vi "SDO_TRAJECTORY_EXECUTE_REL.vi"(8 "Init":bool, 10 "End Relative\nOrientation Deg":dbl, 11 "Gyro Heading\nRAD":dbl) -> (0 "AtReference":bool, 3 "Chassis Velocity Target":T1 {"vOmega" format="%10.3f"; "vY" format="%10.3f"; "vX" format="%10.3f"})   [LabVIEW 2019]
uses:
  <vilib>/Rock Robotics/WPI/ThirdParty/JAS_Junk/TrajLib/Trajectory_Library.lvlib
  PPS_TRAJECTORY_GLOBALS.vi
  <vilib>/Rock Robotics/WPI/ThirdParty/JAS_Junk/TrajLib/TypeDef/CHASSIS_SPEEDS.ctl
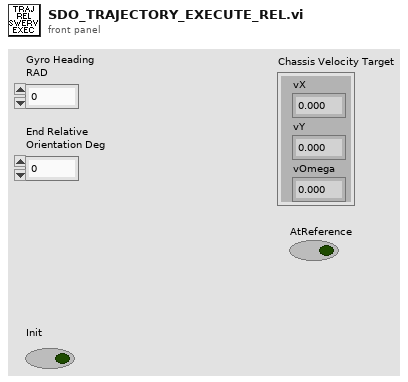
[diagram p1: front panel]
types:
  T1 = typedef "Trajectory_Library.lvlib/CHASSIS_SPEEDS.ctl" = cluster{"vX":dbl, "vY":dbl, "vOmega":dbl}
  T2 = typedef "Trajectory_Library.lvlib/ROTATION2D.ctl" = cluster{"VALUE":dbl, "COS":dbl, "SIN":dbl}
  T3 = typedef "Trajectory_Library.lvlib/SWERVE_DRIVE_KINEMATICS.ctl" = cluster{"NumModules":i32, "InverseKinematics":T4, "ForwardKinematics":T4, "Modules":T5[], "PrevCoR":T5, "SavedModuleStates":T6[]}
  T4 = typedef "NI_Matrix.lvlib/RealMatrix.ctl" = dbl[][]
  T5 = typedef "Trajectory_Library.lvlib/TRANSLATION2D.ctl" = cluster{"X":dbl, "Y":dbl}
  T6 = typedef "Trajectory_Library.lvlib/SWERVE_DRIVE_MODULE_STATE.ctl" = cluster{"Speed":dbl, "Angle":T2}
  T7 = typedef "Trajectory_Library.lvlib/SWERVE_DRIVE_MODULE_POSITION.ctl" = cluster{"Distance":dbl, "Angle":T2, "P":bool}
  T8 = typedef "Trajectory_Library.lvlib/TRAJECTORY.ctl" = cluster{"TotalTImeSecs":dbl, "States":T9[]}
  T9 = typedef "Trajectory_Library.lvlib/TRAJ_STATE.ctl" = cluster{"TimeSeconds":dbl, "Velocity":dbl, "Acceleration":dbl, "POSE":T10, "Curvature":dbl}
  T10 = typedef "Trajectory_Library.lvlib/POSE2D.ctl" = cluster{"TRANSLATION":T5, "ROTATION":T2}
  T11 = typedef "Trajectory_Library.lvlib/PID_TUNING.ctl" = cluster{"Kp":dbl, "Ki":dbl, "Kd":dbl, "MaximumIntegral":dbl, "MinimumIntegral":dbl}
  T12 = typedef "Trajectory_Library.lvlib/PROFILED_PID_CONTROLLER.ctl" = cluster{"Controller":T13, "Goal":T14, "Setpoint":T14, "Constraint":T15}
  T13 = typedef "Trajectory_Library.lvlib/PID_CONTROLLER.ctl" = cluster{"Kp":dbl, "Ki":dbl, "Kd":dbl, "Period":dbl, "Max_Integral":dbl, "Min_Integral":dbl, "Max_Input":dbl, "Min_Input":dbl, "Continuous":bool, "PositionError":dbl, "VelocityError":dbl, "PrevError":dbl, "TotalError":dbl, "PositionTolerance":dbl, "VelocityTolerance":dbl, "SetPoint":dbl, "Kf":dbl, "Prev_Deriv":dbl, "Prev_Deriv 2":dbl, "DerivativeFilter":bool, "Min_Output":dbl, "Max_Output":dbl, "Prev_F_P":dbl, "Prev_F_P_2":dbl, "AntiWindupActive":bool, "Measurement":dbl}
  T14 = typedef "Trajectory_Library.lvlib/TRAPEZOID_PROFILE_STATE.ctl" = cluster{"Position":dbl, "Velocity":dbl}
  T15 = typedef "Trajectory_Library.lvlib/TRAPEZOID_PROFILE_CONSTRAINT.ctl" = cluster{"MaxVelocity":dbl, "MaxAcceleration":dbl}
  T16 = typedef "Trajectory_Library.lvlib/HOLONOMIC_PACK_TUNING.ctl" = cluster{"X PID Tuning":T11, "Y PID Tuning":T11, "thetaProfiledPID_CTRL":T12}
  T17 = typedef "Trajectory_Library.lvlib/HOLONOMIC_DRV_CTRL.ctl" = cluster{"poseTolerance":T10, "poseError":T10, "Enabled":bool, "PID_xCtrl":T13, "PID_yCtrl":T13, "PROF_PID_thetaCtrl":T12, "RotationError":T2, "FirstRun":bool}
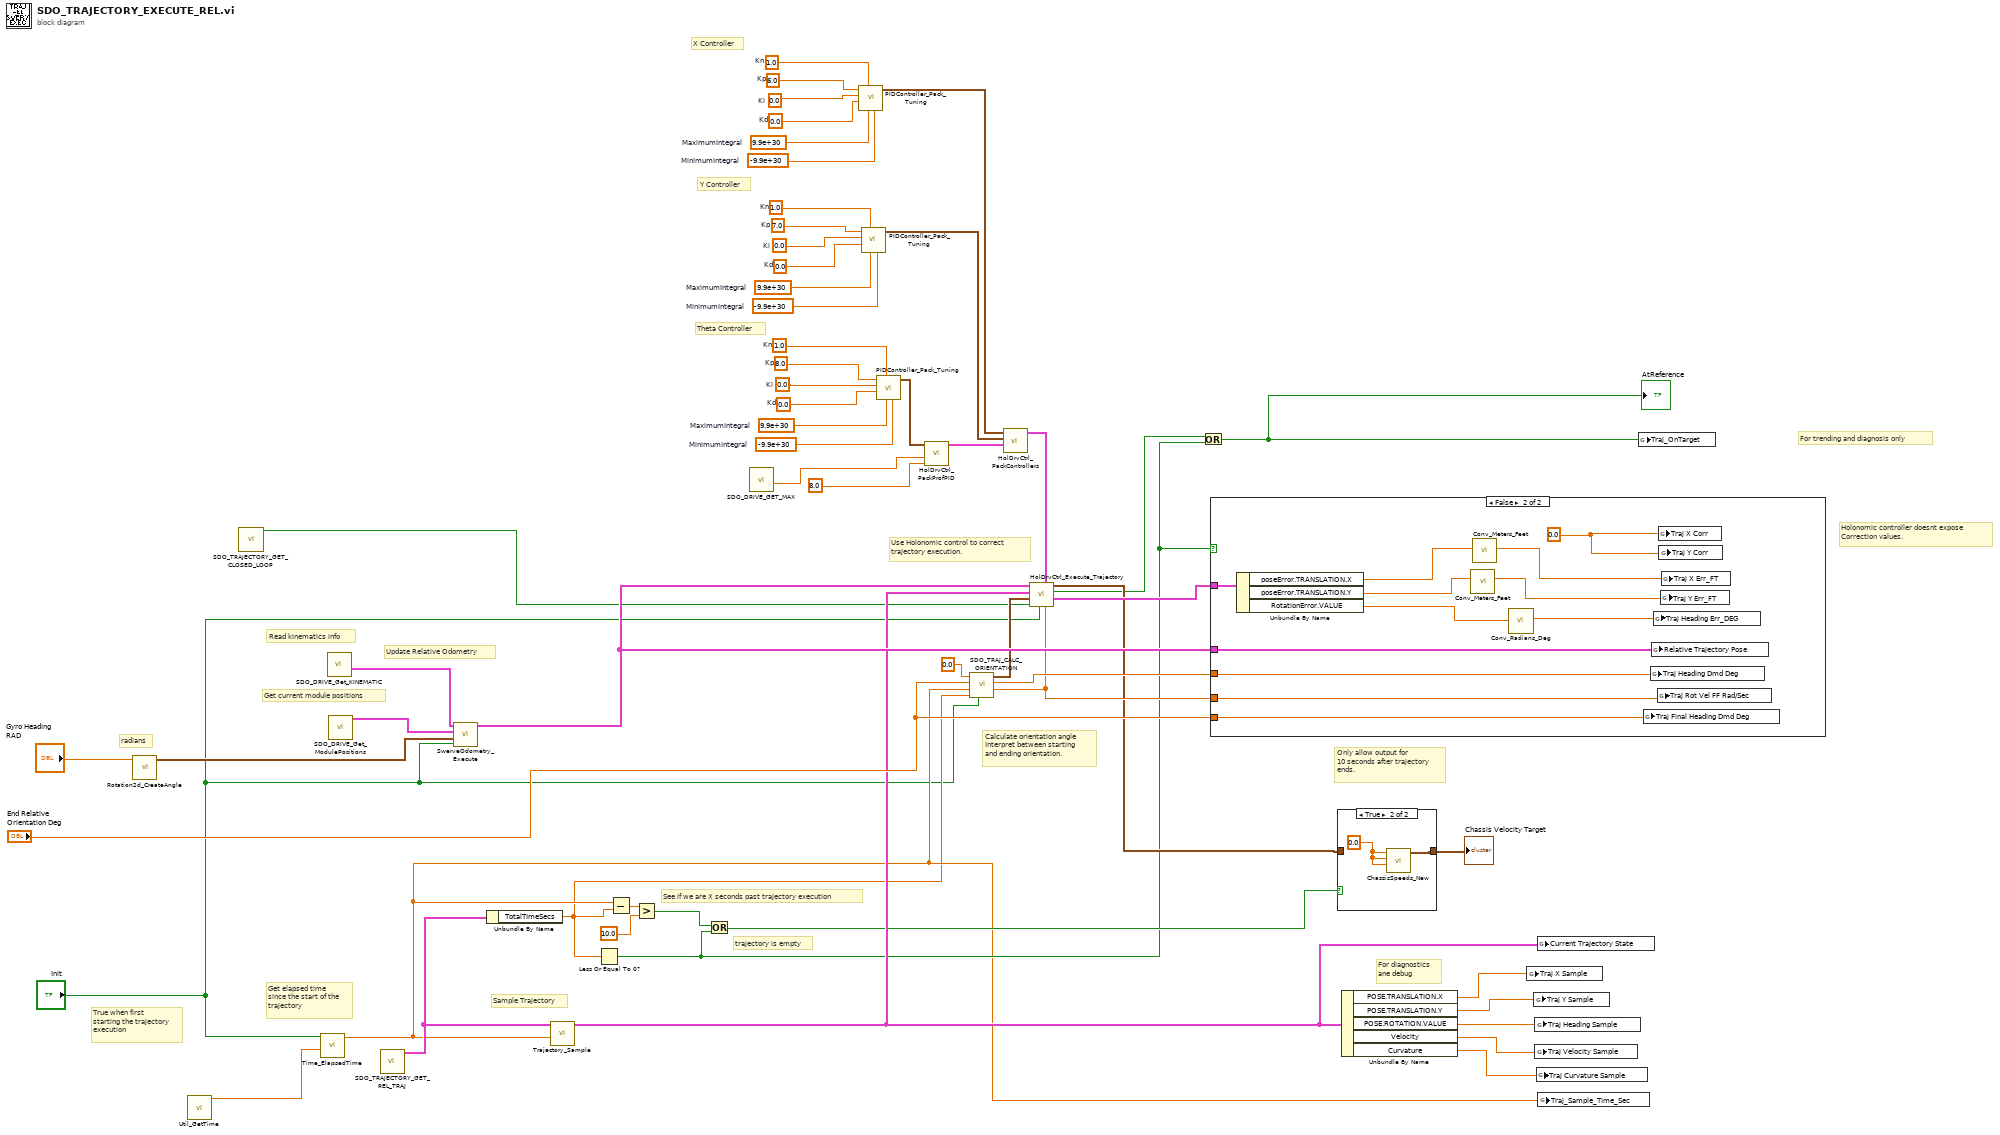
[diagram p0: block diagram]
diagram:
  w24 = 1.0  # Kn
  w27 = 8.0  # Kp
  w36 = 0.0  # Ki
  w37 = 0.0  # Kd
  w38 = 9.9e+30  # MaximumIntegral
  w39 = -9.9e+30  # MinimumIntegral
  w22 = 1.0  # Kn
  w25 = 6.0  # Kp
  w28 = 0.0  # Ki
  w29 = 0.0  # Kd
  w30 = 9.9e+30  # MaximumIntegral
  w31 = -9.9e+30  # MinimumIntegral
  w23 = 1.0  # Kn
  w26 = 7.0  # Kp
  w32 = 0.0  # Ki
  w33 = 0.0  # Kd
  w34 = 9.9e+30  # MaximumIntegral
  w35 = -9.9e+30  # MinimumIntegral
  # "trajectory is empty"
  # "Theta Controller"
  # "Y Controller"
  # "X Controller"
  # "Calculate orientation angle\nInterpret between starting\nand ending orientation."
  # "Get current module positions"
  # "True when first\nstarting the trajectory\nexecution"
  # "Get elapsed time\nsince the start of the\ntrajectory"
  # "Holonomic controller doesnt expose\nCorrection values."
  # "Use Holonomic control to correct\ntrajectory execution."
  # "For trending and diagnosis only"
  # "For diagnostics\nane debug"
  # "Update Relative Odometry"
  # "Read kinematics info"
  # "Sample Trajectory"
  # "See if we are X seconds past trajectory execution"
  # "radians"
  # "Only allow output for\n10 seconds after trajectory\nends."
  n1 = call <vilib>:"Rotation2d_CreateAngle.vi"("Angle"="Gyro Heading\nRAD") -> ("ROTATION"=w53:T2)  [unwired: 10 in]
  n2 = call <vilib>:"Util_GetTime.vi"() -> ("FPGA_Time_Seconds"=w51:dbl)  [unwired: 9 in, 2 out]
  n3 = call "SDO_TRAJECTORY_GET_CLOSED_LOOP.vi"() -> ("AUTO_CLOSED_LOOP"=w1:bool)  [unwired: 11 in]
  n4 = call <vilib>:"Time_ElapsedTime.vi"("PassthroughTime_SEC"=w51, "Reset"="Init") -> ("Elapsed Time Sec"=w4:dbl)  [unwired: 9 in]
  n5 = call "SDO_DRIVE_Get_KINEMATIC.vi"() -> ("out SWERVE_DRIVE_KINEMATICS"=w11:T3)  [unwired: 11 in]
  n6 = call "SDO_DRIVE_Get_ModulePositions.vi"() -> ("Swerve Module Positions"=w52:T7[])  [unwired: 11 in]
  n7 = call "SDO_TRAJECTORY_GET_REL_TRAJ.vi"() -> ("Relative_Trajectory"=w13:T8)  [unwired: 11 in]
  n8 = call <vilib>:"SwerveOdometry_Execute.vi"("Init"="Init", "Rotation"=w53, "Swerve Module Positions"=w52, "SWERVE_DRIVE_KINEMATICS"=w11) -> ("Current Pose"=w20:T10)  [unwired: 5 in, 2 out]
  n9 = Unbundle By Name(w13) -> ("TotalTImeSecs"=w3:dbl)
  n10 = call <vilib>:"Trajectory_Sample.vi"("Time"=w4, "InputTRAJECTORY"=w13) -> ("OutputTRAJ_STATE"=w12:T9)  [unwired: 9 in]
  n11 = Less Or Equal To 0?(x=w3) -> (x <= 0?=w5:bool)
  n12 = Subtract(x=w4, y=w3) -> (x-y=w57:dbl)
  n13 = Greater?(x=w57, y=10.0) -> (0:w9:bool)
  n14 = Or(x=w9, y=w5) -> (x .or. y?=w8:bool)
  n15 = call "SDO_DRIVE_GET_MAX.vi"() -> ("Max Rotational Vel (Rad/Sec)"=w15:dbl)  [unwired: 10 in, 1 out]
  n16 = call <vilib>:"PIDController_Pack_Tuning.vi"("MinimumIntegral"=w31, "MaximumIntegral"=w30, "Kn"=w22, "Kd"=w29, "Ki"=w28, "Kp"=w25) -> ("PID Tuning"=w40:T11)  [unwired: 5 in]
  n17 = call <vilib>:"PIDController_Pack_Tuning.vi"("MinimumIntegral"=w35, "MaximumIntegral"=w34, "Kn"=w23, "Kd"=w33, "Ki"=w32, "Kp"=w26) -> ("PID Tuning"=w41:T11)  [unwired: 5 in]
  n18 = call <vilib>:"PIDController_Pack_Tuning.vi"("MinimumIntegral"=w39, "MaximumIntegral"=w38, "Kn"=w24, "Kd"=w37, "Ki"=w36, "Kp"=w27) -> ("PID Tuning"=w21:T11)  [unwired: 5 in]
  n19 = call <vilib>:"HolDrvCtrl_PackProfPID.vi"("Max Accel"=8.0, "Max Speed"=w15, "Theta PID Tuning"=w21) -> ("Theta PID CONTROLLER"=w42:T12)  [unwired: 8 in]
  n20 = call "SDO_TRAJ_CALC_ORIENTATION.vi"("Init"="Init", "Total Trajectory Time Sec"=w3, "Elapsed Traj Time Sec"=w4, "End Orientation Demand DEG"="End Relative\nOrientation Deg", "Starting Orientation  DEG"=0.0) -> ("Rotational Velocity Rad Per Sec"=w17:dbl, "Orientation Demand Deg"=w45:dbl, "Orientation Demand"=w19:T2)  [unwired: 4 in]
  n21 = call <vilib>:"HolDrvCtrl_PackControllers.vi"("thetaProfiledPID_CTRL"=w42, "Y PID Tuning"=w41, "X PID Tuning"=w40) -> ("HOLONOMIC_CTRL_PACK_TUNING"=w43:T16)  [unwired: 8 in]
  n22 = call <vilib>:"HolDrvCtrl_Execute_Trajectory.vi"("Rotational Velocity Feedforward \nRad/Sec"=w17, "HOLONOMIC_CTRL_PACK_TUNING"=w43, "Reset"="Init", "Enable"=w1, "angleRef"=w19, "desiredTrajState"=w12, "currentPose"=w20) -> ("outHOLONOMIC_DRV_CTRL"=w18:T17, "AtReference"=w7:bool, "calcChassisSpeed"=w10:T1)  [unwired: 2 in]
  n23 = Or(x=w7, y=w5) -> (x .or. y?=w6:bool)
  "AtReference" <- w6
  n24 = case shown="False" w5 {
    tunnel: w45 -> [_ w68]
    tunnel: "End Relative\nOrientation Deg" -> [_ w67]
    tunnel: w20 -> [_ w61]
    tunnel: w18 -> [_ w60]
    tunnel: w17 -> [_ w59]
    frame True {
    }
    frame False {
      w69 = 0.0 ("Y Corr")
      n25 = Unbundle By Name(w60) -> ("poseError.TRANSLATION.X"=w65:dbl, "poseError.TRANSLATION.Y"=w64:dbl, "RotationError.VALUE"=w58:dbl)
      n26 = call <vilib>:"Conv_Meters_Feet.vi"("Meters"=w64) -> ("Feet"=w63:dbl)  [unwired: 10 in]
      n27 = call <vilib>:"Conv_Meters_Feet.vi"("Meters"=w65) -> ("Feet"=w62:dbl)  [unwired: 10 in]
      n28 = call <vilib>:"Conv_Radians_Deg.vi"("Radians"=w58) -> ("Degrees"=w66:dbl)  [unwired: 10 in]
      n29 = global write "PPS_TRAJECTORY_GLOBALS.vi" "Traj Final Heading Dmd Deg"(w67) -> ()
      n30 = global write "PPS_TRAJECTORY_GLOBALS.vi" "Traj Heading Dmd Deg"(w68) -> ()
      n31 = global write "PPS_TRAJECTORY_GLOBALS.vi" "Relative Trajectory Pose"(w61) -> ()
      n32 = global write "PPS_TRAJECTORY_GLOBALS.vi" "Traj Heading Err_DEG"(w66) -> ()
      n33 = global write "PPS_TRAJECTORY_GLOBALS.vi" "Traj Rot Vel FF Rad/Sec"(w59) -> ()
      n34 = global write "PPS_TRAJECTORY_GLOBALS.vi" "Traj X Corr"(w69) -> ()
      n35 = global write "PPS_TRAJECTORY_GLOBALS.vi" "Traj Y Corr"(w69) -> ()
      n36 = global write "PPS_TRAJECTORY_GLOBALS.vi" "Traj Y Err_FT"(w63) -> ()
      n37 = global write "PPS_TRAJECTORY_GLOBALS.vi" "Traj X Err_FT"(w62) -> ()
    }
  }
  n38 = case shown="True" w8 {
    tunnel: w10 -> [w70 _]
    tunnel: [w70 w71] -> w54
    frame False {
    }
    frame True {
      w72 = 0.0 ("vX")
      n39 = call <vilib>:"ChassisSpeeds_New.vi"("vAngular"=w72, "vY"=w72, "vX"=w72) -> ("CHASSIS"=w71:T1)  [unwired: 8 in]
    }
  }
  "Chassis Velocity Target" <- w54
  n40 = Unbundle By Name(w12) -> ("POSE.TRANSLATION.X"=w50:dbl, "POSE.TRANSLATION.Y"=w49:dbl, "POSE.ROTATION.VALUE"=w48:dbl, "Velocity"=w47:dbl, "Curvature"=w46:dbl)
  n41 = global write "PPS_TRAJECTORY_GLOBALS.vi" "Traj X Sample"(w50) -> ()
  n42 = global write "PPS_TRAJECTORY_GLOBALS.vi" "Traj Y Sample"(w49) -> ()
  n43 = global write "PPS_TRAJECTORY_GLOBALS.vi" "Traj Heading Sample"(w48) -> ()
  n44 = global write "PPS_TRAJECTORY_GLOBALS.vi" "Traj Velocity Sample"(w47) -> ()
  n45 = global write "PPS_TRAJECTORY_GLOBALS.vi" "Traj Curvature Sample"(w46) -> ()
  n46 = global write "PPS_TRAJECTORY_GLOBALS.vi" "Current Trajectory State"(w12) -> ()
  n47 = global write "PPS_TRAJECTORY_GLOBALS.vi" "Traj_Sample_Time_Sec"(w4) -> ()
  n48 = global write "PPS_TRAJECTORY_GLOBALS.vi" "Traj_OnTarget"(w6) -> ()
